vi "showCell.vi"(11 "Cell in":refnum<class "Cell.lvclass">) -> (0 "AdjacentMines":dbl, 1 "hasFlag":bool, 2 "isMine":bool, 3 "isCovered":bool, 4 "Column index":dbl, 5 "Line index":dbl)   [LabVIEW 2014, in "Cell.lvclass"]
uses:
  Cell.lvclass
  Cell.lvclass/Cell.ctl
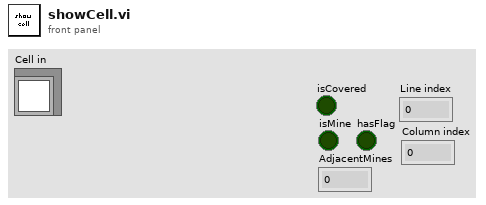
[diagram p1: front panel]
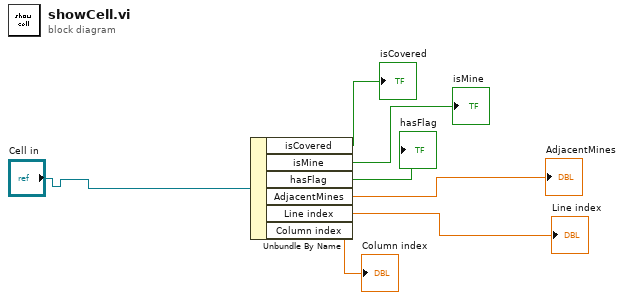
[diagram p0: block diagram]
diagram:
  n1 = Unbundle By Name("Cell in") -> ("isCovered"=→"isCovered":bool, "isMine"=→"isMine":bool, "hasFlag"=→"hasFlag":bool, "AdjacentMines"=→"AdjacentMines":dbl, "Line index"=→"Line index":dbl, "Column index"=→"Column index":dbl)
